vi "Handle WebSocket Upgrade.vi"(8 "error in (no error)":errorcluster, 10 "Response.lvclass":refnum<class "Response.lvclass">, 11 "Request.lvclass":refnum<class "Request.lvclass">) -> (0 "error out":errorcluster, 3 "WebSocket":refnum<class "WebSocket.lvclass">)   [LabVIEW 2023]
doc: "Use this template to build a VI to use as a subVI."
uses:
  Request/Request.lvclass
  Response/Response.lvclass
  WebSocket/WebSocket.lvclass
  Request/Get Request.vi
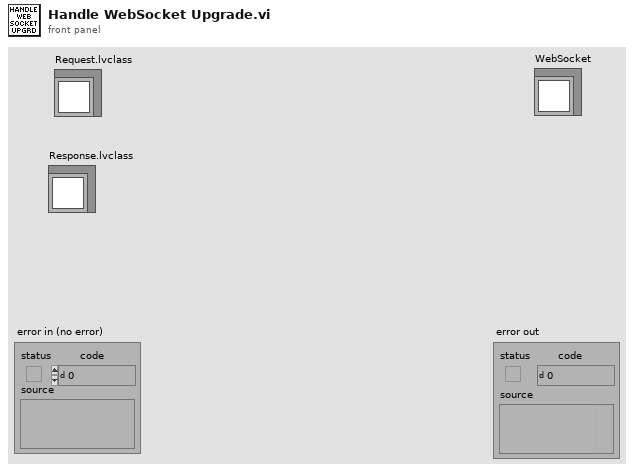
[diagram p1: front panel]
types:
  T1 = typedef "Request.ctl" = cluster{"Method":string, "URI":string, "Protocol":string, "Raw Path":string, "Query":string, "Fragment":string, "Raw Body":string, "Headers":variant, "Parameters":variant, "Body":variant, "Raw Header":string, "Path":string[]}
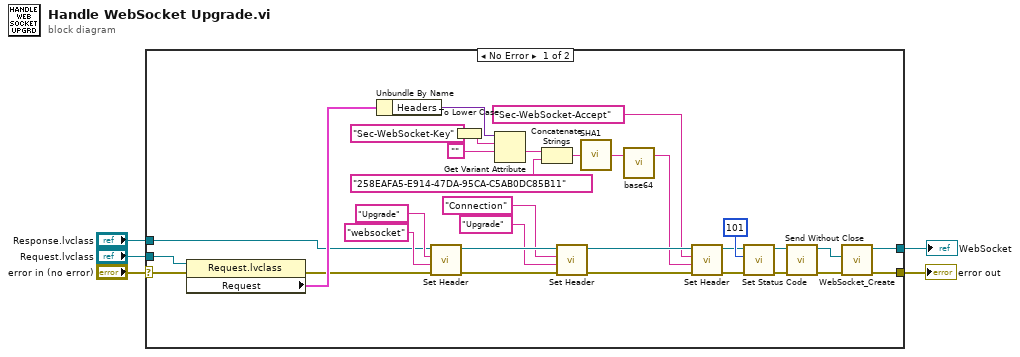
[diagram p0: block diagram]
diagram:
  n1 = case shown="No Error" "error in (no error)" {
    selector: "error in (no error)" -> [w11 w38]
    tunnel: [w7 w38] -> w4
    tunnel: "Request.lvclass" -> [w9 _]
    tunnel: "Response.lvclass" -> [w8 _]
    tunnel: [w6 _] -> w1
    frame No Error {
      n2 = property class="Request.lvclass"(reference=w9, error in=w11) -> (error out=w10:errorcluster, "Request"=w12:T1)  [unwired: 1 out]
      n3 = Unbundle By Name(w12) -> ("Headers"=w13:variant)
      n4 = call "Set Header.vi"("error in (no error)"=w10, "Value"="websocket", "Header"="Upgrade", "Response in"=w8) -> ("error out"=w28:errorcluster, "Response out"=w34:refnum<class "Response.lvclass">)  [unwired: 5 in, 1 out]
      n5 = To Lower Case(string="Sec-WebSocket-Key" ("trimmed string")) -> (all lower case string=w14:string)
      n6 = Get Variant Attribute(Variant=w13, name=w14, default value (empty Variant)="") -> (value=w22:string)  [unwired: 1 in, 3 out]
      n7 = Concatenate Strings(w22, "258EAFA5-E914-47DA-95CA-C5AB0DC85B11" ("trimmed string")) -> (w23:string)
      n8 = call "Set Header.vi"("error in (no error)"=w28, "Value"="Upgrade", "Header"="Connection", "Response in"=w34) -> ("error out"=w27:errorcluster, "Response out"=w33:refnum<class "Response.lvclass">)  [unwired: 5 in, 1 out]
      n9 = call "SHA1.vi"("String"=w23) -> ("SHA1"=w24:string)
      n10 = call "base64.vi"("string in"=w24) -> ("base64 out"=w19:string)  [unwired: 1 in, 1 out]
      n11 = call "Set Header.vi"("error in (no error)"=w27, "Value"=w19, "Header"="Sec-WebSocket-Accept", "Response in"=w33) -> ("error out"=w17:errorcluster, "Response out"=w18:refnum<class "Response.lvclass">)  [unwired: 5 in, 1 out]
      n12 = call "Set Status Code.vi"("error in (no error)"=w17, "Status Code"=u16 101, "Response in"=w18) -> ("error out"=w36:errorcluster, "Response out"=w37:refnum<class "Response.lvclass">)  [unwired: 7 in]
      n13 = call "Send Without Close.vi"("error in (no error)"=w36, "Response in"=w37) -> ("error out"=w15:errorcluster, "connection ID out"=w16:refnum<k5>)  [unwired: 8 in]
      n14 = call "WebSocket_Create.vi"("error in (no error)"=w15, "Socket"=w16) -> ("error out"=w7:errorcluster, "reference out"=w6:refnum<class "WebSocket.lvclass">)  [unwired: 8 in]
    }
    frame Error {
    }
  }
  "error out" <- w4
  "WebSocket" <- w1
